vi "FPGA_MAIN.vi"   [LabVIEW 2016]
uses:
  <vilib>/rvi/Emulation/niFpgaSctlEmulationGetInTimedLoop.vi
  Global 1.vi
  <vilib>/rvi/Emulation/niFpgaProcessEmulError.vi
  <vilib>/rvi/Emulation/niFpgaGetClockAttributes.vi
  <vilib>/rvi/Emulation/niFpgaEmulationReportErrorSimple.vi
  <vilib>/rvi/eio/common/nirviEmuTemplateMethod_errors.vi
  <vilib>/rvi/Emulation/niFpgaCriticalErrorInLSC.vi
  <vilib>/eio/EIONode/EIONode.xnode
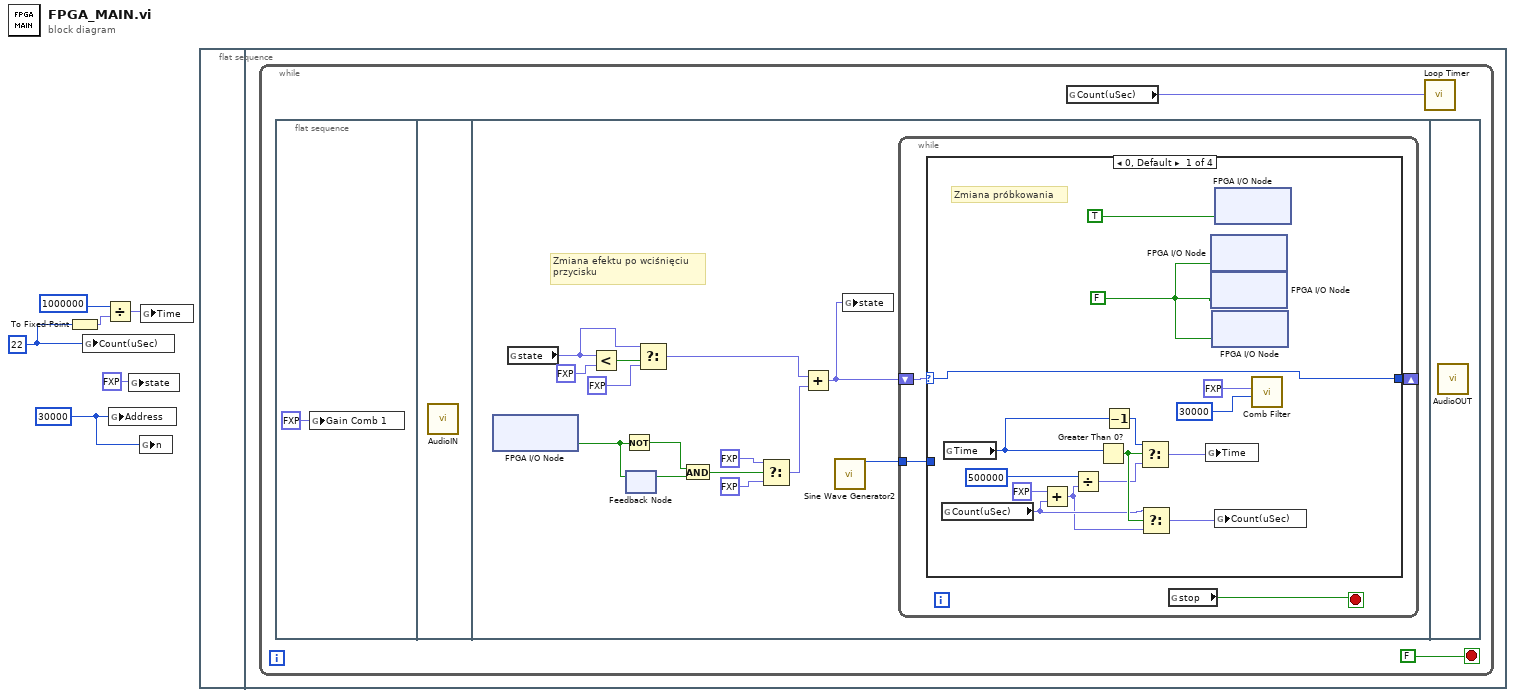
[diagram p0: block diagram]
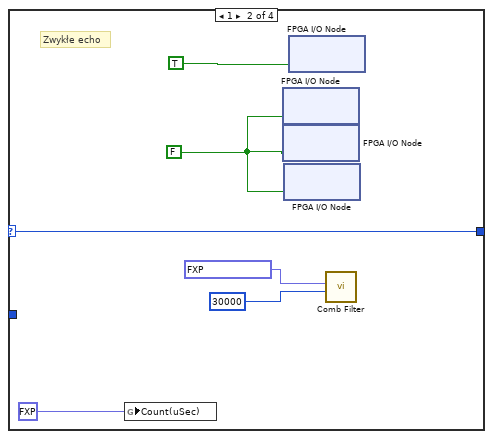
[diagram p2: hidden frame]
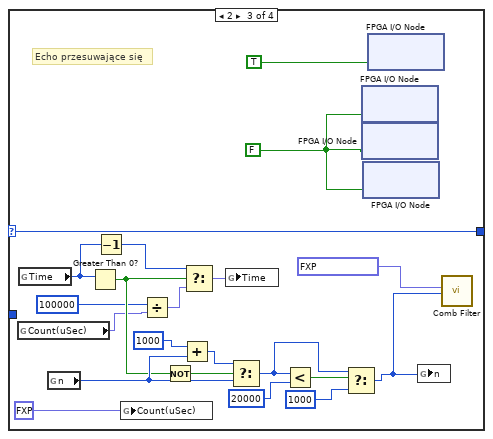
[diagram p3: hidden frame]
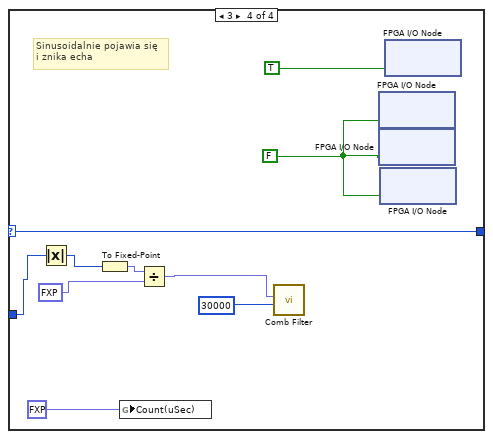
[diagram p4: hidden frame]
diagram:
  w1 = 30000 ("n")
  w2 = u32 22 ("Count(uSec) 2")
  n1 = To Fixed-Point(number=w2) -> (fixed-point=w4:fxp<+,32,32>)  [unwired: 1 in]
  n2 = global write "Global 1.vi" "Count(uSec)"(w2) -> ()
  n3 = Divide(x=u32 1000000, y=w4) -> (x/y=w6:fxp<+,64,32>)
  n4 = global write "Global 1.vi" "Address"(w1) -> ()
  n5 = global write "Global 1.vi" "state"(fxp<+/-,25,16> 0.0 ("state")) -> ()
  n6 = global write "Global 1.vi" "n"(w1) -> ()
  n7 = global write "Global 1.vi" "Time"(w6) -> ()
  n8 = flat-sequence {
    frame #0 {
    }
    frame #1 {
      n9 = while {
        stop <- FALSE stop-if-true
        n10 = flat-sequence {
          frame #0 {
            n11 = global write "Global 1.vi" "Gain Comb 1"(fxp<+/-,25,16> 1.0 ("Gain Comb 1")) -> ()
          }
          frame #1 {
            n12 = call "AudioIN.vi"() -> ()  [unwired: 12 in]
          }
          frame #2 {
            # "Zmiana efektu po wciśnięciu\nprzycisku"
            n13 = xnode "FPGA I/O Node"() -> ("Button0"=w15:bool)  [unwired: 1 in, 1 out]
            n14 = global read "Global 1.vi" "state"() -> (w21:fxp<+/-,25,16>)
            n15 = Less?(x=w21, y=fxp<+/-,25,16> 4.0) -> (x < y?=w22:bool)
            n16 = Not(x=w15) -> (.not. x?=w13:bool)
            n17 = feedback-in #1(w15) -> ()
            n18 = feedback #1() -> (w14:bool)  [unwired: 1 in]
            n19 = Select(t=w21, s=w22, f=fxp<+/-,25,16> -1.0) -> (s? t:f=w16:fxp<+/-,25,16>)
            n20 = And(x=w13, y=w14) -> (x .and. y?=w12:bool)
            n21 = Select(t=fxp<+,1,1> 1.0, s=w12, f=fxp<+,1,1> 0.0) -> (s? t:f=w17:fxp<+,1,1>)
            n22 = Add(x=w16, y=w17) -> (x+y=w10:fxp<+/-,26,17>)
            n23 = call "Sine Wave Generator2"() -> ("sine out"=w11:i8)  [unwired: 15 in]
            n24 = global write "Global 1.vi" "state"(w10) -> ()
            n25 = while {
              shift-right: [w25] -> _
              shift-left: w10 -> [w26]
              tunnel: w11 -> [w24]
              stop <- w27 stop-if-true
              n26 = case shown="0, Default" w26 {
                selector: w26 -> [w29 w46 w67 w77]
                tunnel: [w29 w46 w67 w77] -> w25
                tunnel: w24 -> [_ _ _ w74]
                frame 0, Default {
                  w41 = FALSE ("LED0")
                  # "Zmiana próbkowania"
                  n27 = global read "Global 1.vi" "Count(uSec)"() -> (w33:fxp<+/-,25,16>)
                  n28 = global read "Global 1.vi" "Time"() -> (w38:u32)
                  n29 = Add(x=fxp<+/-,25,16> 20.0, y=w33) -> (x+y=w30:fxp<+/-,26,17>)
                  n30 = Divide(x=u32 500000, y=w30) -> (x/y=w32:fxp<+/-,59,42>)
                  n31 = Greater Than 0?(x=w38) -> (x > 0?=w34:bool)
                  n32 = Decrement(x=w38) -> (x-1=w37:u32)
                  n33 = Select(t=w37, s=w34, f=w32) -> (s? t:f=w39:fxp<+/-,59,42>)
                  n34 = Select(t=w33, s=w34, f=w30) -> (s? t:f=w31:fxp<+/-,26,17>)
                  n35 = global write "Global 1.vi" "Time"(w39) -> ()
                  n36 = xnode "FPGA I/O Node"("LED1"=w41) -> ()  [unwired: 1 in, 1 out]
                  n37 = xnode "FPGA I/O Node"("LED2"=w41) -> ()  [unwired: 1 in, 1 out]
                  n38 = xnode "FPGA I/O Node"("LED3"=w41) -> ()  [unwired: 1 in, 1 out]
                  n39 = xnode "FPGA I/O Node"("LED0"=TRUE) -> ()  [unwired: 1 in, 1 out]
                  n40 = global write "Global 1.vi" "Count(uSec)"(w31) -> ()
                  n41 = call "Comb Filter.vi"("n"=i64 30000, "g"=fxp<+/-,16,4> 0.0) -> ()  [unwired: 3 in]
                }
                frame 1 {
                  w47 = FALSE ("LED0")
                  # "Zwykłe echo"
                  n42 = global write "Global 1.vi" "Count(uSec)"(fxp<+/-,25,16> 22.0 ("Count(uSec)")) -> ()
                  n43 = xnode "FPGA I/O Node"("LED0"=w47) -> ()  [unwired: 1 in, 1 out]
                  n44 = xnode "FPGA I/O Node"("LED2"=w47) -> ()  [unwired: 1 in, 1 out]
                  n45 = xnode "FPGA I/O Node"("LED3"=w47) -> ()  [unwired: 1 in, 1 out]
                  n46 = xnode "FPGA I/O Node"("LED1"=TRUE ("LED0")) -> ()  [unwired: 1 in, 1 out]
                  n47 = call "Comb Filter.vi"("n"=i64 30000, "g"=fxp<+/-,16,4> 0.800048828125) -> ()  [unwired: 3 in]
                }
                frame 2 {
                  w68 = FALSE ("LED0")
                  # "Echo przesuwające się"
                  n48 = global read "Global 1.vi" "Count(uSec)"() -> (w50:fxp<+/-,25,16>)
                  n49 = global read "Global 1.vi" "Time"() -> (w64:u32)
                  n50 = global read "Global 1.vi" "n"() -> (w62:i64)
                  n51 = Greater Than 0?(x=w64) -> (x > 0?=w54:bool)
                  n52 = Decrement(x=w64) -> (x-1=w63:u32)
                  n53 = global write "Global 1.vi" "Count(uSec)"(fxp<+/-,25,16> 22.0 ("Count(uSec)")) -> ()
                  n54 = Divide(x=u32 100000, y=w50) -> (x/y=w49:fxp<+/-,58,42>)
                  n55 = Not(x=w54) -> (.not. x?=w53:bool)
                  n56 = Add(x=i64 1000, y=w62) -> (x+y=w60:i64)
                  n57 = Select(t=w63, s=w54, f=w49) -> (s? t:f=w65:fxp<+/-,58,42>)
                  n58 = global write "Global 1.vi" "Time"(w65) -> ()
                  n59 = Select(t=w60, s=w53, f=w62) -> (s? t:f=w57:i64)
                  n60 = Less?(x=w57, y=i64 20000) -> (x < y?=w58:bool)
                  n61 = Select(t=w57, s=w58, f=i64 1000) -> (s? t:f=w56:i64)
                  n62 = xnode "FPGA I/O Node"("LED0"=w68) -> ()  [unwired: 1 in, 1 out]
                  n63 = xnode "FPGA I/O Node"("LED1"=w68) -> ()  [unwired: 1 in, 1 out]
                  n64 = xnode "FPGA I/O Node"("LED3"=w68) -> ()  [unwired: 1 in, 1 out]
                  n65 = xnode "FPGA I/O Node"("LED2"=TRUE ("LED0")) -> ()  [unwired: 1 in, 1 out]
                  n66 = global write "Global 1.vi" "n"(w56) -> ()
                  n67 = call "Comb Filter.vi"("n"=w56, "g"=fxp<+/-,16,4> 0.89990234375) -> ()  [unwired: 3 in]
                }
                frame 3 {
                  w78 = FALSE ("LED0")
                  # "Sinusoidalnie pojawia się\ni znika echa"
                  n68 = Absolute Value(x=w74) -> (abs(x)=w71:i8)
                  n69 = To Fixed-Point(number=w71) -> (fixed-point=w72:fxp<+/-,8,8>)  [unwired: 1 in]
                  n70 = global write "Global 1.vi" "Count(uSec)"(fxp<+/-,25,16> 22.0 ("Count(uSec)")) -> ()
                  n71 = Divide(x=w72, y=fxp<+,16,7> 100.0) -> (x/y=w75:fxp<+/-,32,16>)
                  n72 = call "Comb Filter.vi"("n"=i64 30000, "g"=w75) -> ()  [unwired: 3 in]
                  n73 = xnode "FPGA I/O Node"("LED0"=w78) -> ()  [unwired: 1 in, 1 out]
                  n74 = xnode "FPGA I/O Node"("LED1"=w78) -> ()  [unwired: 1 in, 1 out]
                  n75 = xnode "FPGA I/O Node"("LED2"=w78) -> ()  [unwired: 1 in, 1 out]
                  n76 = xnode "FPGA I/O Node"("LED3"=TRUE ("LED0")) -> ()  [unwired: 1 in, 1 out]
                }
              }
              n77 = global read "Global 1.vi" "stop"() -> (w27:bool)
            }
          }
          frame #3 {
            n78 = call "AudioOUT.vi"() -> ()  [unwired: 12 in]
          }
        }
        n79 = global read "Global 1.vi" "Count(uSec)"() -> (w7:fxp<+/-,25,16>)
        n80 = call "Loop Timer"("Count(uSec)"=w7) -> ()  [unwired: 1 out]
      }
    }
  }
